vi "Update.vi"(8 "error in (no error)":errorcluster, 11 "Dual Fan in":refnum<class "Dual Fan.lvclass">) -> (0 "error out":errorcluster, 3 "Dual Fan out":refnum<class "Dual Fan.lvclass">)   [LabVIEW 2012, in "Dual Fan.lvlib" / "Dual Fan.lvclass"]
uses:
  Dual Fan.lvclass
  Simulation/Simulation Data_Global.vi
  Simulation/Simulation.lvlib
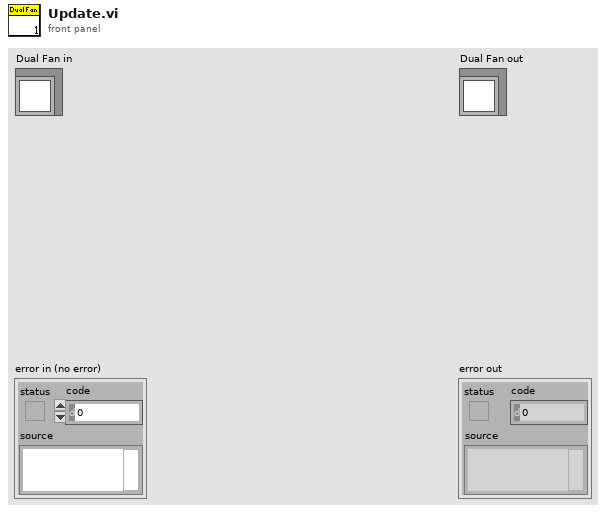
[diagram p1: front panel]
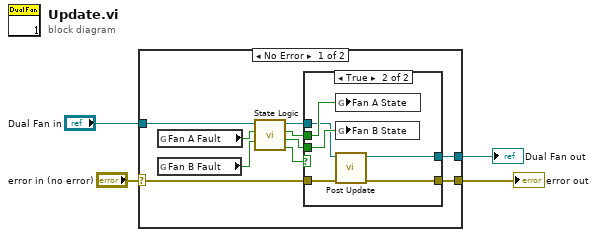
[diagram p0: block diagram]
diagram:
  n1 = case shown="No Error" "error in (no error)" {
    selector: "error in (no error)" -> [w6 w24]
    tunnel: [w5 w24] -> w3
    tunnel: "Dual Fan in" -> [w14 w23]
    tunnel: [w11 w23] -> w1
    frame No Error {
      n2 = global read "Simulation Data_Global.vi" "Fan A Fault"() -> (w9:bool)
      n3 = global read "Simulation Data_Global.vi" "Fan B Fault"() -> (w10:bool)
      n4 = call "State Logic.vi"("Fan B Fault"=w10, "Fan A Fault"=w9, "Dual Fan in"=w14) -> ("State Changed"=w13:bool, "Fan B State"=w7:bool, "Fan A State"=w8:bool, "Dual Fan out"=w12:refnum<class "Dual Fan.lvclass">)  [unwired: 5 in]
      n5 = case shown="True" w13 {
        tunnel: w12 -> [w16 w19]
        tunnel: [w16 w18] -> w11
        tunnel: w8 -> [_ w22]
        tunnel: w7 -> [_ w21]
        tunnel: w6 -> [w15 w20]
        tunnel: [w15 w17] -> w5
        frame False {
        }
        frame True {
          n6 = global write "Simulation Data_Global.vi" "Fan A State"(w22) -> ()
          n7 = global write "Simulation Data_Global.vi" "Fan B State"(w21) -> ()
          n8 = call "Post Update.vi"("error in (no error)"=w20, "Dual Fan in"=w19) -> ("error out"=w17:errorcluster, "Dual Fan out"=w18:refnum<class "Dual Fan.lvclass">)  [unwired: 8 in]
        }
      }
    }
    frame Error {
    }
  }
  "error out" <- w3
  "Dual Fan out" <- w1
